vi "Write XML.vi"(8 "error in (no error)":errorcluster, 10 "String":string, 11 "Configuration in":refnum<class "Configuration.lvclass">) -> (0 "error out":errorcluster, 3 "Configuration out":refnum<class "Configuration.lvclass">)   [LabVIEW 2011, in "Configuration.lvclass"]
uses:
  Configuration.lvclass
  Configuration.lvclass/Configuration.ctl
  <vilib>/Utility/xml.llb/Write to XML File(string).vi
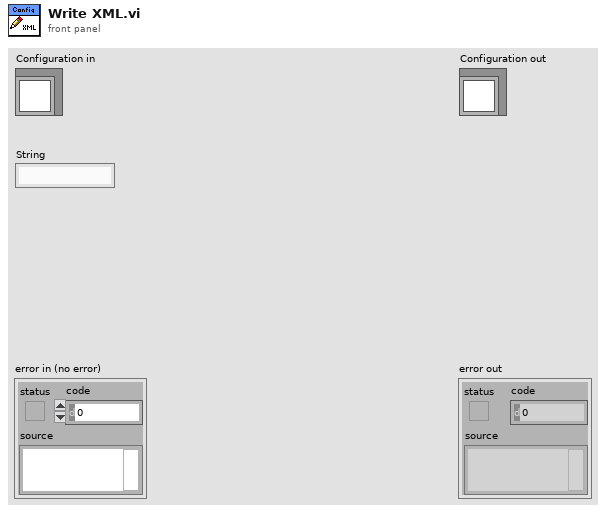
[diagram p1: front panel]
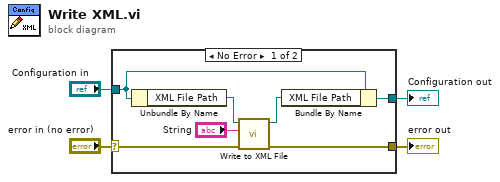
[diagram p0: block diagram]
diagram:
  n1 = case shown="No Error" "error in (no error)" {
    selector: "error in (no error)" -> [w8 w13]
    tunnel: [w7 w13] -> w3
    tunnel: [w5 w12] -> w1
    tunnel: "Configuration in" -> [w10 w12]
    frame No Error {
      n2 = Unbundle By Name(w10) -> ("XML File Path"=w11:path)
      n3 = call-poly <vilib>:"Write to XML File.vi"("error in (no error)"=w8, "XML Input"="String", "XML File Path"=w11) -> ("error out"=w7:errorcluster, "XML File Path(duplicate)"=w9:path)  [unwired: 2 in, 5 out]
      n4 = Bundle By Name(cluster=w10, "XML File Path"=w9) -> (w5:refnum<class "Configuration.lvclass">)
    }
    frame Error {
    }
  }
  "error out" <- w3
  "Configuration out" <- w1
